vi "Reports.Report Config - Read.vi"(6 "Default Rpt Dir":path=path "c:/MTE/Results", 7 "Config File":path, 8 "error in (no error)":errorcluster, 9 "Dialog":bool, 10 "Save Only":bool, 11 "Report Config In":T1[](array[typedef])) -> (0 "error out":errorcluster, 3 "Report Config Out":T1[](array[typedef]))   [LabVIEW 2019]
uses:
  Report.Report File Config Item.ctl
  Report.Report File Type.ctl
  <vilib>/KATE/Files/File Utils.lvlib
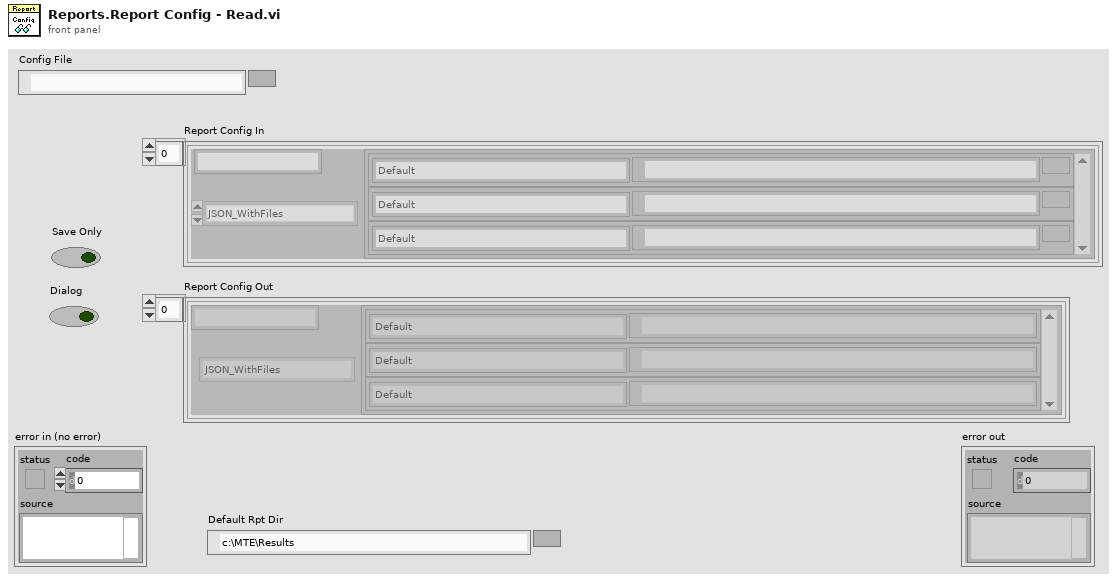
[diagram p1: front panel]
types:
  T1 = typedef "Report.Report File Config Item.ctl" = cluster{"Name":string, "Type":T2, "Seq_Dir":cluster{"Sequence":string, "Folder":path}[]}
  T2 = typedef "Report.Report File Type.ctl" = enum16{"CSV_WithConfigAndData", "CSV", "CSV_SummaryResult", "JSON", "JSON_WithFiles", "XLINK", "XLINK_ResultOnly", "SFC1", ""}
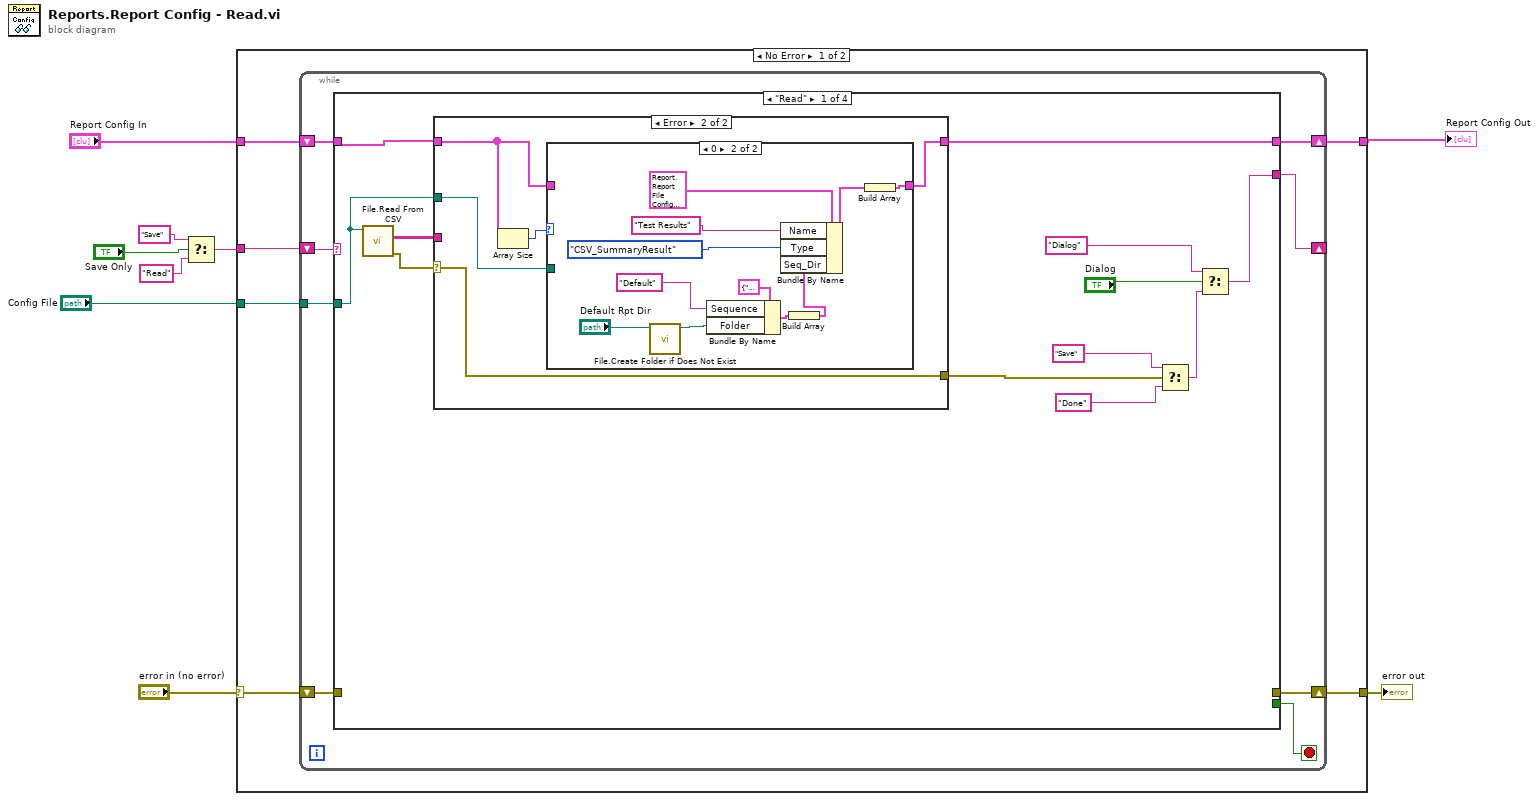
[diagram p0: block diagram]
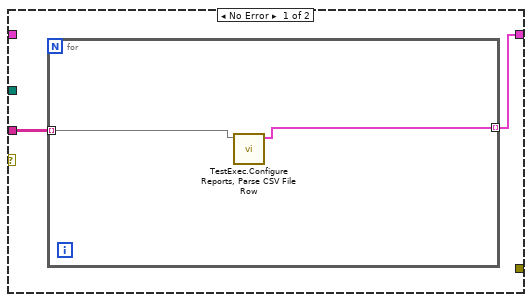
[diagram p2: hidden frame]
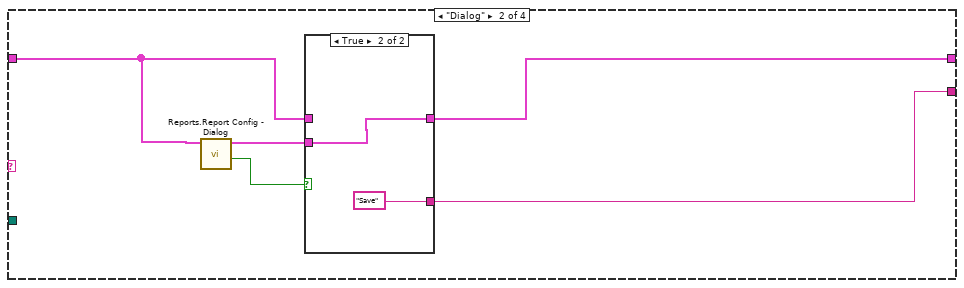
[diagram p4: hidden frame]
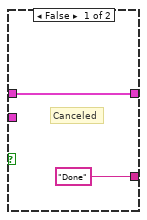
[diagram p5: hidden frame]
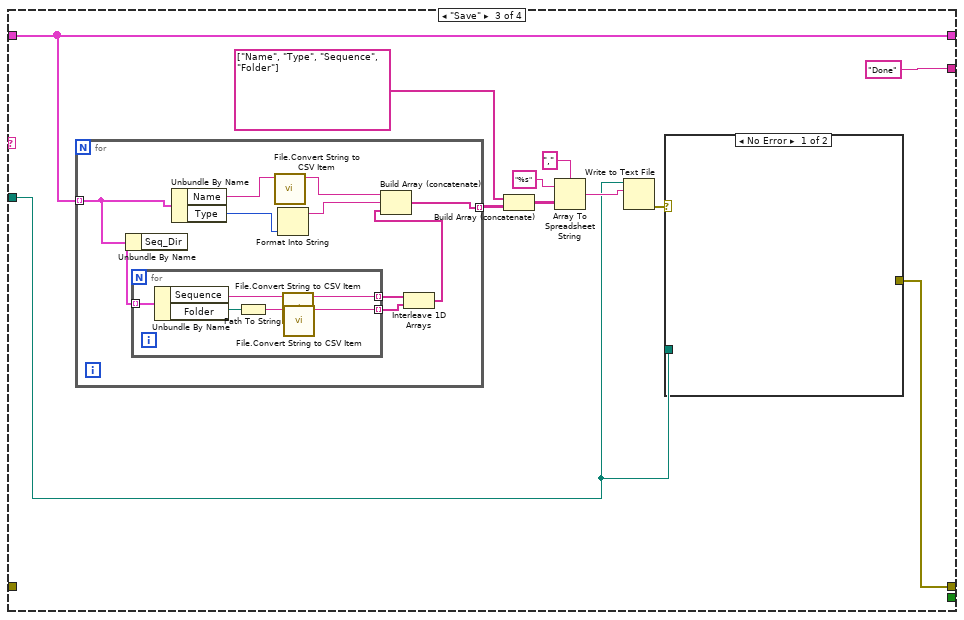
[diagram p6: hidden frame]
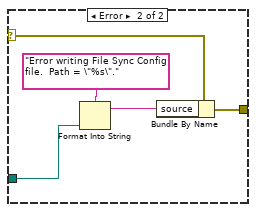
[diagram p7: hidden frame]
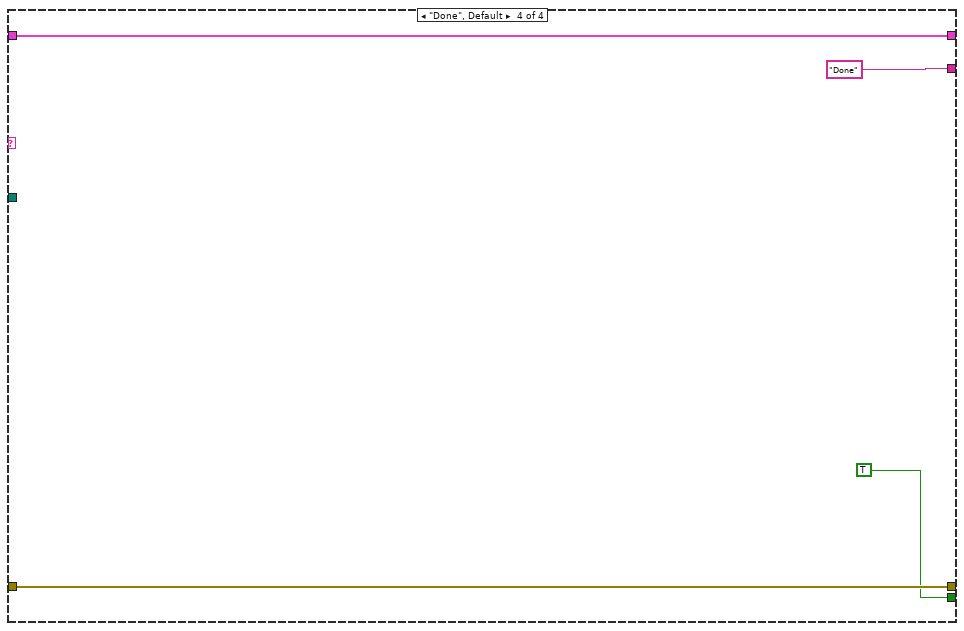
[diagram p8: hidden frame]
diagram:
  n1 = Select(t="Save", s="Save Only", f="Read") -> (s? t:f=w3:string)
  n2 = case shown="No Error" "error in (no error)" {
    selector: "error in (no error)" -> [w13 w103]
    tunnel: [w12 w103] -> w8
    tunnel: [w14 w102] -> w1
    tunnel: "Report Config In" -> [w10 w102]
    tunnel: "Config File" -> [w15 _]
    tunnel: w3 -> [w11 _]
    frame No Error {
      n3 = while {
        tunnel: w15 -> [w23]
        shift-right: [w21] -> w14
        shift-left: w10 -> [w22]
        shift-right: [w18] -> _
        shift-left: w11 -> [w19]
        shift-right: [w17] -> w12
        shift-left: w13 -> [w20]
        stop <- w16 stop-if-true
        n4 = case shown="\"Read\"" w19 {
          tunnel: w23 -> [w26 _ w68 _]
          tunnel: w22 -> [w25 w57 w66 w101]
          tunnel: [w31 w59 w66 w101] -> w21
          tunnel: w20 -> [_ _ _ w99]
          tunnel: [w32 w58 "Done" "Done"] -> w18
          tunnel: [_ _ w67 w99] -> w17
          tunnel: [_ _ _ TRUE] -> w16
          frame "Read" {
            n5 = call <vilib>:"File.Read From CSV.vi"("File"=w26) -> ("error out"=w30:errorcluster, "Data"=w35:string[][])  [unwired: 8 in, 1 out]
            n6 = case shown="Error" w30 {
              selector: w30 -> [_ w44]
              tunnel: w35 -> [w37 _]
              tunnel: [w36 w41] -> w31
              tunnel: w25 -> [_ w42]
              tunnel: [_ w44] -> w24
              tunnel: w26 -> [_ w40]
              frame No Error {
                n7 = for {
                  tunnel: w37 -> [w39] mode=indexing
                  tunnel: [w38] -> w36 mode=indexing
                  n8 = call "TestExec.Configure Reports, Parse CSV File Row.vi"("Array"=w39) -> ("Report Config Item"=w38:T1)  [unwired: 10 in]
                }
              }
              frame Error {
                n9 = Array Size(array=w42) -> (size(s)=w43:i32)
                n10 = case shown="0" w43 {
                  tunnel: w42 -> [w45 _]
                  tunnel: [w45 w56] -> w41
                  tunnel: w40 -> [_ _]
                  frame Default {
                  }
                  frame 0 {
                    n11 = call <vilib>:"File.Create Folder if Does Not Exist.vi"("Path"="Default Rpt Dir") -> ("Dup Path"=w46:path)  [unwired: 8 in, 2 out]
                    n12 = Bundle By Name(cluster=cluster{"Sequence":string, "Folder":path} {"Sequence"="", "Folder"=path ""} ("Cluster"), "Sequence"="Default", "Folder"=w46) -> (w50:cluster{"Sequence":string, "Folder":path})
                    n13 = Build Array(w50) -> (w49:cluster{"Sequence":string, "Folder":path}[])
                    n14 = Bundle By Name(cluster=T1 {"Name"="", "Type"=enum."CSV_WithConfigAndData", "Seq_Dir"=[]} ("Report Config Item"), "Name"="Test Results", "Type"=Report.Report_File_Type."CSV_SummaryResult", "Seq_Dir"=w49) -> (w54:T1)
                    n15 = Build Array(w54) -> (w56:T1[])
                  }
                }
              }
            }
            n16 = Select(t="Save", s=w24, f="Done") -> (s? t:f=w27:string)
            n17 = Select(t="Dialog", s="Dialog", f=w27) -> (s? t:f=w32:string)
          }
          frame "Dialog" {
            n18 = call "Reports.Report Config - Dialog.vi"("Report Config"=w57) -> ("OK"=w61:bool, "Report Config Out"=w60:T1[])  [unwired: 9 in]
            n19 = case shown="True" w61 {
              tunnel: w60 -> [_ w64]
              tunnel: w57 -> [w63 _]
              tunnel: [w63 w64] -> w59
              tunnel: ["Done" "Save"] -> w58
              frame False {
                # "Canceled"
              }
              frame True {
              }
            }
          }
          frame "Save" {
            n20 = for {
              tunnel: w66 -> [w86] mode=indexing
              tunnel: [w91] -> w74 mode=indexing
              n21 = Unbundle By Name(w86) -> ("Seq_Dir"=w85:cluster{"Sequence":string, "Folder":path}[])
              n22 = for {
                tunnel: w85 -> [w96] mode=indexing
                tunnel: [w93] -> w84 mode=indexing
                tunnel: [w92] -> w83 mode=indexing
                n23 = Unbundle By Name(w96) -> ("Sequence"=w94:string, "Folder"=w95:path)
                n24 = Path To String(path=w95) -> (string=w97:string)
                n25 = call <vilib>:"File.Convert String to CSV Item.vi"("String"=w94) -> ("String Out"=w93:string)  [unwired: 10 in]
                n26 = call <vilib>:"File.Convert String to CSV Item.vi"("String"=w97) -> ("String Out"=w92:string)  [unwired: 10 in]
              }
              n27 = Unbundle By Name(w86) -> ("Name"=w90:string, "Type"=w88:T2)
              n28 = call <vilib>:"File.Convert String to CSV Item.vi"("String"=w90) -> ("String Out"=w89:string)  [unwired: 10 in]
              n29 = Format Into String(w88) -> (resulting string=w87:string)  [unwired: 3 in, 1 out]
              n30 = Interleave 1D Arrays(w84, w83) -> (w82:string[])
              n31 = Build Array (concatenate)(w89, w87, w82) -> (w91:string[])
            }
            n32 = Build Array (concatenate)(string[] ["Name", "Type", "Sequence", "Folder"], w74) -> (w73:string[][])
            n33 = Array To Spreadsheet String(delimiter (Tab)=",", array=w73, 3:"%s" ("format string")) -> (spreadsheet string=w70:string)
            n34 = Write to Text File(file (use dialog)=w68, text=w70) -> (error out=w69:errorcluster)  [unwired: 2 in, 2 out]
            n35 = case shown="No Error" w69 {
              selector: w69 -> [_ w81]
              tunnel: w68 -> [_ w78]
              tunnel: [_ w80] -> w67
              frame No Error {
              }
              frame Error {
                n36 = Format Into String(format string="Error writing File Sync Config file.  Path = \"%s\".", w78) -> (resulting string=w77:string)  [unwired: 2 in, 1 out]
                n37 = Bundle By Name(cluster=w81, "source"=w77) -> (w80:errorcluster)
              }
            }
          }
          frame "Done", Default {
          }
        }
      }
    }
    frame Error {
    }
  }
  "error out" <- w8
  "Report Config Out" <- w1
